vi "Get ProjectItem Descendants.vi"(8 "error in (no error)":errorcluster, 11 "ProjectItem in":refnum<vi>) -> (0 "error out":errorcluster, 2 "All Descendents":refnum<vi>[](array[refnum]), 3 "ProjectItem out":refnum<vi>)   [LabVIEW 2019, in "gRPC Template Creation Utility.lvlib"]
uses:
  gRPC Template Creation Utility.lvlib
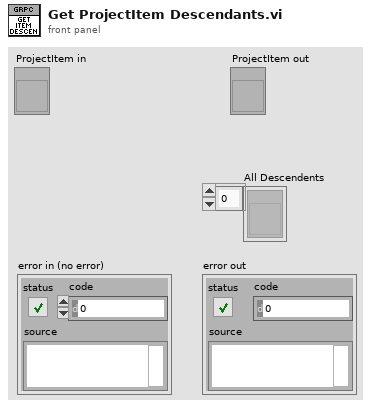
[diagram p1: front panel]
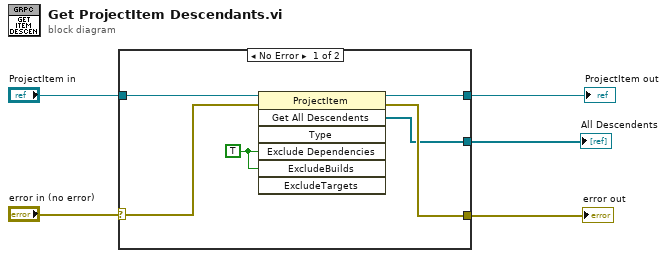
[diagram p0: block diagram]
diagram:
  n1 = case shown="No Error" "error in (no error)" {
    selector: "error in (no error)" -> [w7 w12]
    tunnel: "ProjectItem in" -> [w11 w13]
    tunnel: [w9 w12] -> w4
    tunnel: [w8 _] -> w3
    tunnel: [w6 w13] -> w1
    frame No Error {
      w10 = TRUE ("ExcludeDependencies")
      n2 = invoke class="ProjectItem" method="Get All Descendents"(reference=w11, error in=w7, "Exclude Dependencies"=w10, "ExcludeBuilds"=w10) -> (reference out=w6:refnum<vi>, error out=w9:errorcluster, "All Descendents"=w8:refnum<vi>[])  [unwired: 3 in, 4 out]
    }
    frame Error {
    }
  }
  "error out" <- w4
  "All Descendents" <- w3
  "ProjectItem out" <- w1
